vi "Review Recipe for Overlap.vi"(6 "Waypoints":cluster{"x":dbl, "y":dbl, "th":dbl}[](array[cluster]), 8 "Blends":T1[](array[typedef]), 11 "Min R":dbl[](array[numeric])) -> (0 "Blends out":T1[](array[typedef]), 2 "Linear Info":T2(array[cluster]), 3 "Length (f)":dbl, 4 "Waypoints out":cluster{"x":dbl, "y":dbl, "th":dbl}[](array[cluster]))   [LabVIEW 2019]
uses:
  BlendType.ctl
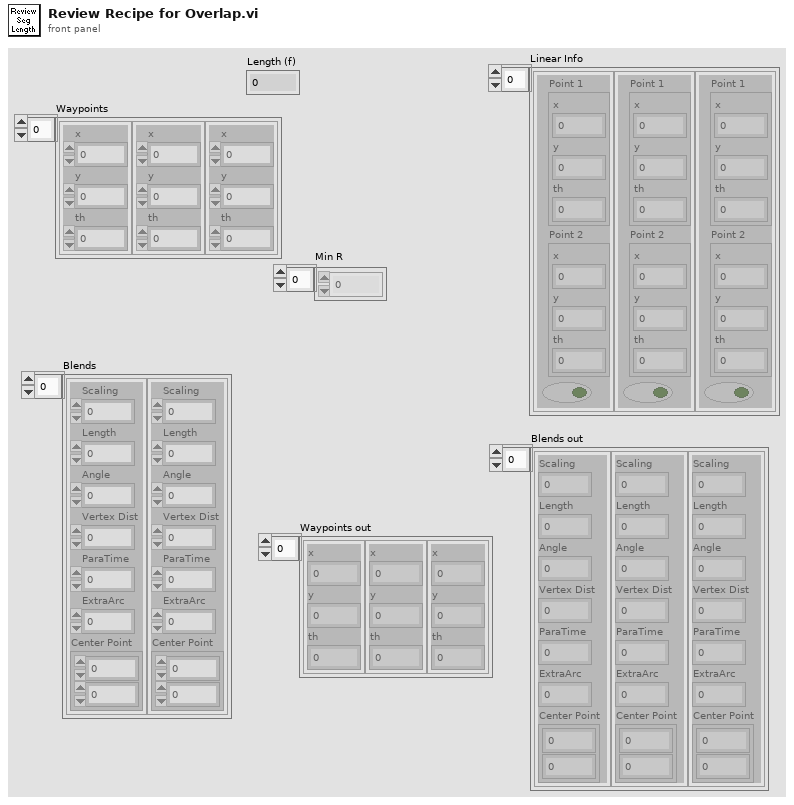
[diagram p1: front panel]
types:
  T1 = typedef "BlendType.ctl" = cluster{"Scaling":dbl, "Length":dbl, "Angle":dbl, "Vertex Dist":dbl, "ParaTime":dbl, "ExtraArc":dbl, "Center Point":cluster{dbl, dbl}}
  T2 = cluster{"Point 1":cluster{"x":dbl, "y":dbl, "th":dbl}, "Point 2":cluster{"x":dbl, "y":dbl, "th":dbl}, bool}[]
  T3 = cluster{"Point Out":cluster{"x":dbl, "y":dbl, "th":dbl}, "Point Out":cluster{"x":dbl, "y":dbl, "th":dbl}, bool}
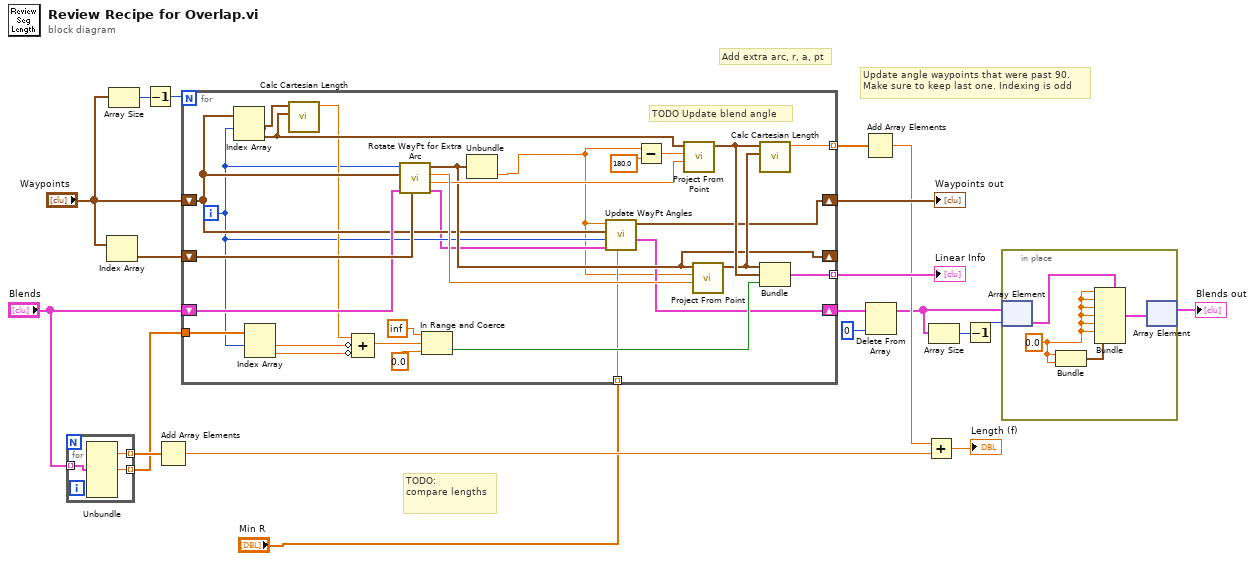
[diagram p0: block diagram]
diagram:
  # "TODO:\ncompare lengths"
  # "Update angle waypoints that were past 90.\nMake sure to keep last one. Indexing is odd"
  # "Add extra arc, r, a, pt"
  n1 = for {
    tunnel: "Blends" -> [w23] mode=indexing
    tunnel: [w22] -> w10 mode=indexing
    tunnel: [w21] -> w9 mode=indexing
    n2 = Unbundle(w23) -> ("Length"=w22:dbl, "Vertex Dist"=w21:dbl)  [unwired: 5 out]
  }
  n3 = Index Array(array="Waypoints") -> (element=w16:cluster{"x":dbl, "y":dbl, "th":dbl})  [unwired: 1 in]
  n4 = Array Size(array="Waypoints") -> (size(s)=w12:i32)
  n5 = Decrement(x=w12) -> (x-1=w13:i32)
  n6 = Add Array Elements(numeric array=w10) -> (sum=w8:dbl)
  n7 = for {
    N: w13 -> [_]
    tunnel: [w51] -> w19 mode=indexing
    tunnel: [w46] -> w20 mode=indexing
    shift-right: [w41] -> _
    shift-left: w16 -> [w45]
    shift-right: [w26] -> w18
    shift-left: "Blends" -> [w44]
    shift-right: [w39] -> w15
    shift-left: "Waypoints" -> [w40]
    tunnel: w9 -> [w38]
    tunnel: "Min R" -> [w25] mode=indexing
    i -> [w28]
    # "TODO Update blend angle"
    n8 = Index Array(array=w40, index #1=w28) -> (element #1=w37:cluster{"x":dbl, "y":dbl, "th":dbl}, element #2=w36:cluster{"x":dbl, "y":dbl, "th":dbl})  [unwired: 1 in]
    n9 = Index Array(array=w38, index #1=w28) -> (element #1=w33:dbl, element #2=w34:dbl)  [unwired: 1 in]
    n10 = call "Calc Cartesian Length.vi"("Point 2"=w36, "Point 1"=w37) -> ("Length (f)"=w35:dbl)  [unwired: 8 in, 1 out]
    n11 = Compound Arithmetic op=ADD(w35, invert w33, invert w34) -> (w32:dbl)
    n12 = call "Rotate WayPt for Extra Arc.vi"("Pt 0"=w45, "Blends In"=w44, "Pts"=w40, "index"=w28) -> ("Blends Out"=w27:T1[], "Pt2 vertex dist"=w42:dbl, "Pt0 vertex dist"=w43:dbl, "Pt Out"=w41:cluster{"x":dbl, "y":dbl, "th":dbl})  [unwired: 4 in]
    n13 = In Range and Coerce(upper limit=inf, x=w32, lower limit=0.0 ("upper limit")) -> (In Range?=w29:bool)  [unwired: 1 out]
    n14 = Unbundle(w41) -> ("th"=w24:dbl)  [unwired: 2 out]
    n15 = call "Update WayPt Angles.vi"("Min R"=w25, "Blends In"=w27, "Index"=w28, "Waypoints in"=w40, "th"=w24) -> ("Blends Out"=w26:T1[], "Waypoints out"=w39:cluster{"x":dbl, "y":dbl, "th":dbl}[])  [unwired: 5 in]
    n16 = Subtract(x=w24, y=180.0) -> (x-y=w50:dbl)
    n17 = call "Project From Point.vi"("distance"=w42, "th"=w50, "Point In"=w36) -> ("Point Out"=w48:cluster{"x":dbl, "y":dbl, "th":dbl})  [unwired: 8 in]
    n18 = call "Project From Point.vi"("distance"=w43, "th"=w24, "Point In"=w41) -> ("Point Out"=w47:cluster{"x":dbl, "y":dbl, "th":dbl})  [unwired: 8 in]
    n19 = call "Calc Cartesian Length.vi"("Point 2"=w47, "Point 1"=w48) -> ("Length (f)"=w46:dbl)  [unwired: 8 in, 1 out]
    n20 = Bundle("Point Out"=w47, "Point Out"=w48, w29) -> (w51:T3)  [unwired: 1 in]
  }
  "Linear Info" <- w19
  "Waypoints out" <- w15
  n21 = Add Array Elements(numeric array=w20) -> (sum=w7:dbl)
  n22 = Delete From Array(array=w18, index=0) -> (array with subset deleted=w4:T1[])  [unwired: 1 in, 1 out]
  n23 = Add(x=w7, y=w8) -> (x+y=→"Length (f)":dbl)
  n24 = Array Size(array=w4) -> (size(s)=w3:i32)
  n25 = Decrement(x=w3) -> (x-1=w2:i32)
  n26 = in-place {
    w53 = 0.0 ("ExtraArc")
    n27 = in-place-array #1(w4, w2) -> (w55:T1)
    n28 = Bundle("ExtraArc"=w53, "ExtraArc"=w53) -> (w52:cluster{"ExtraArc":dbl, "ExtraArc":dbl})  [unwired: 1 in]
    n29 = Bundle(cluster=w55, "Scaling"=w53, "Length"=w53, "Angle"=w53, "Vertex Dist"=w53, "ParaTime"=w53, "ExtraArc"=w53, "Center Point"=w52) -> (w54:T1)
    n30 = in-place-array #1(w54) -> (→"Blends out":T1[])  [unwired: 1 out]
  }
